vi "Create Results Directory.vi"(8 "error in":errorcluster, 11 "Peer Review in":refnum<class "Peer Review.lvclass">) -> (0 "error out":errorcluster, 3 "Peer Review out":refnum<class "Peer Review.lvclass">)   [LabVIEW 2020, in "Peer Review.lvclass"]
uses:
  Peer Review.lvclass
  Peer Review.lvclass/Peer Review.ctl
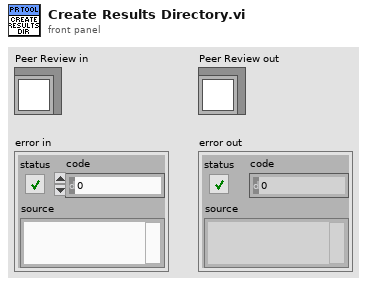
[diagram p1: front panel]
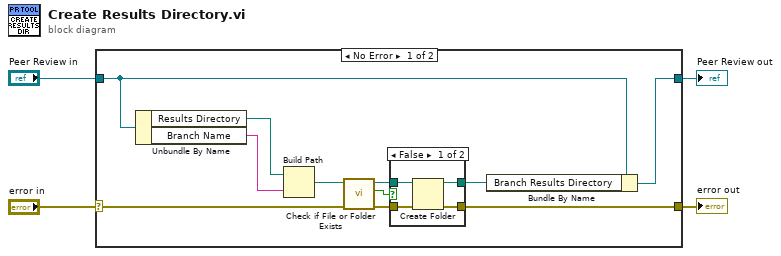
[diagram p0: block diagram]
diagram:
  n1 = case shown="No Error" "error in" {
    selector: "error in" -> [w5 w22]
    tunnel: [w15 w23] -> w4
    tunnel: [w11 w22] -> w2
    tunnel: "Peer Review in" -> [w8 w23]
    frame No Error {
      n2 = Unbundle By Name(w8) -> ("Results Directory"=w14:path, "Branch Name"=w6:string)
      n3 = Build Path(base path=w14, name or relative path=w6) -> (appended path=w12:path)
      n4 = call <vilib>:"Check if File or Folder Exists.vi"("error in (no error)"=w5, "path"=w12) -> ("error out"=w9:errorcluster, "file or folder exists?"=w7:bool, "dup path"=w10:path)  [unwired: 7 in]
      n5 = case shown="False" w7 {
        tunnel: [w17 w21] -> w11
        tunnel: w9 -> [w19 w21]
        tunnel: w10 -> [w18 w20]
        tunnel: [w16 w20] -> w13
        frame False {
          n6 = Create Folder(path (use dialog)=w18, error in=w19) -> (created path=w16:path, error out=w17:errorcluster)  [unwired: 1 in, 1 out]
        }
        frame True {
        }
      }
      n7 = Bundle By Name(cluster=w8, "Branch Results Directory"=w13) -> (w15:refnum<class "Peer Review.lvclass">)
    }
    frame Error {
    }
  }
  "Peer Review out" <- w4
  "error out" <- w2
